vi "ShiftRegisterTutorial.vi"() -> ()   [LabVIEW 2018]
panel:
  out "Value of Sum":i32
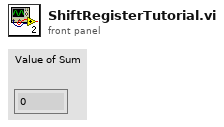
[diagram p1: front panel]
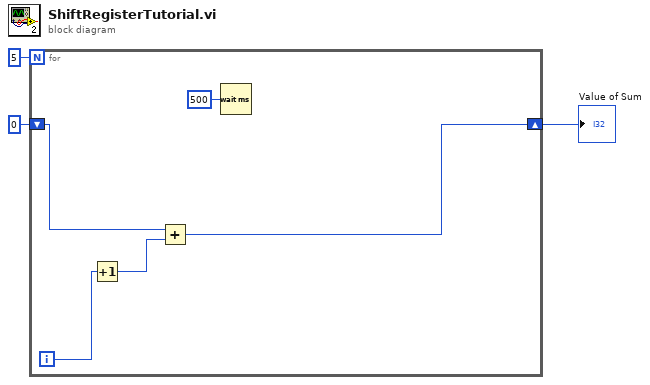
[diagram p0: block diagram]
diagram:
  n1 = for {
    N: 5 -> [_]
    shift-right: [w6] -> w2
    shift-left: 0 -> [w5]
    i -> [w7]
    n2 = Increment(x=w7) -> (x+1=w8:i32)
    n3 = Add(x=w5, y=w8) -> (x+y=w6:i32)
    n4 = Wait (ms)(milliseconds to wait=u32 500) -> ()  [unwired: 1 out]
  }
  "Value of Sum" <- w2
